vi "Util_CreateNIDrop.vi"(8 "error in (no error)":errorcluster) -> (0 "error out":errorcluster)   [LabVIEW 2011]
doc: "Runs the embedded application on a console located in the <B>Build Path</B> directory ."
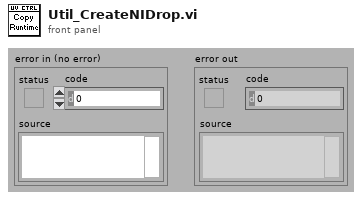
[diagram p1: front panel]
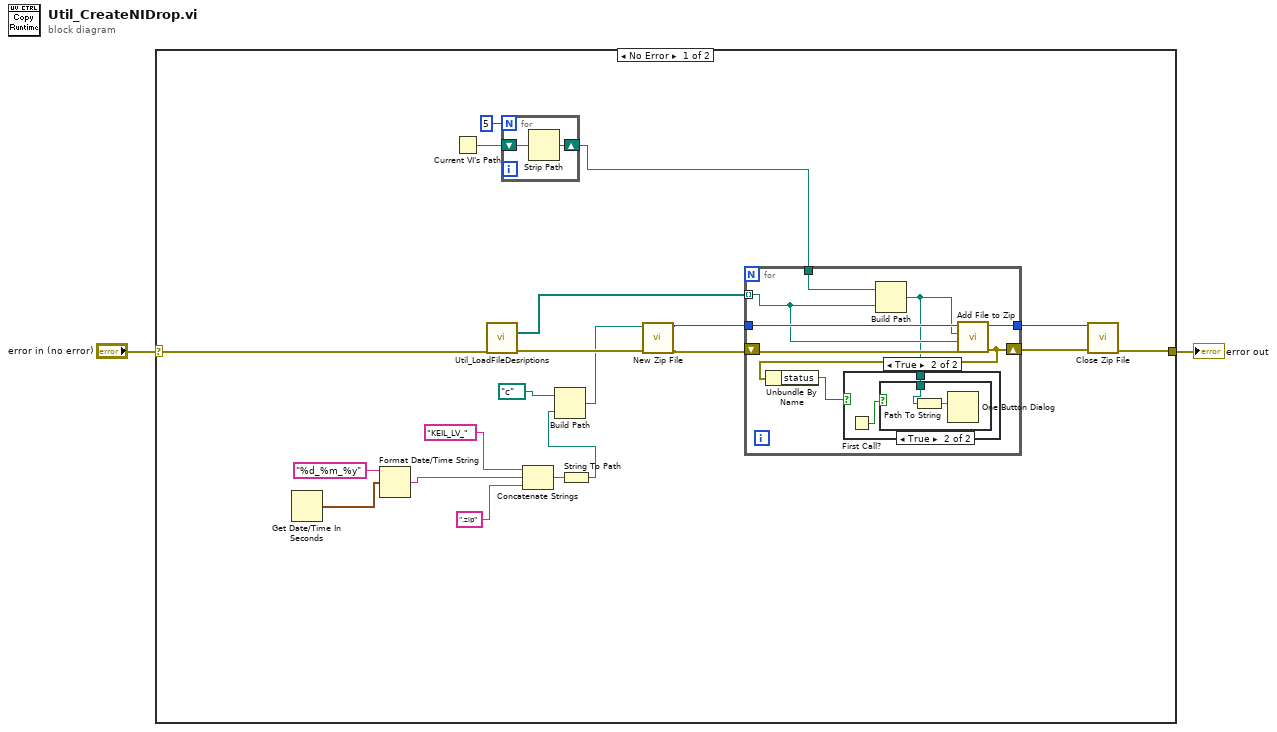
[diagram p0: block diagram]
diagram:
  n1 = case shown="No Error" "error in (no error)" {
    selector: "error in (no error)" -> [w16 w37]
    tunnel: [w10 w37] -> w1
    frame No Error {
      n2 = Get Date/Time In Seconds() -> (seconds since 1Jan1904=w22:timestamp)
      n3 = Format Date/Time String(time format string (%c)="%d_%m_%y", seconds (now)=w22) -> (date/time string=w8:string)  [unwired: 1 in]
      n4 = Current VI's Path() -> (path=w15:path)
      n5 = call "Util_LoadFileDesriptions.vi"("error in (no error)"=w16) -> ("Drop Files"=w17:path[], "error out"=w20:errorcluster)  [unwired: 9 in, 4 out]
      n6 = for {
        N: 5 -> [_]
        shift-right: [w23] -> w13
        shift-left: w15 -> [w24]
        n7 = Strip Path(path=w24) -> (stripped path=w23:path)  [unwired: 1 out]
      }
      n8 = Concatenate Strings("KEIL_LV_", w8, ".zip") -> (w6:string)
      n9 = String To Path(string=w6) -> (path=w3:path)
      n10 = Build Path(base path=path "c:/", name or relative path=w3) -> (appended path=w4:path)
      n11 = call <vilib>:"New Zip File.vi"("error in (no error)"=w20, "target"=w4) -> ("error out"=w19:errorcluster, "zip file out"=w18:i64)  [unwired: 3 in, 1 out]
      n12 = for {
        tunnel: w18 -> [w32]
        tunnel: w17 -> [w30] mode=indexing
        shift-right: [w27] -> w12
        shift-left: w19 -> [w31]
        tunnel: w13 -> [w29]
        tunnel: [w28] -> w11
        n13 = Build Path(base path=w29, name or relative path=w30) -> (appended path=w25:path)
        n14 = call <vilib>:"Add File to Zip.vi"("error in (no error)"=w31, "destination path in zip"=w30, "source file path"=w25, "zip file in"=w32) -> ("error out"=w27:errorcluster, "zip file out"=w28:i64)  [unwired: 6 in]
        n15 = Unbundle By Name(w27) -> ("status"=w26:bool)
        n16 = case shown="True" w26 {
          tunnel: w25 -> [_ w33]
          frame False {
          }
          frame True {
            n17 = First Call?() -> (First Call?: T/F=w34:bool)
            n18 = case shown="True" w34 {
              tunnel: w33 -> [_ w35]
              frame False {
              }
              frame True {
                n19 = Path To String(path=w35) -> (string=w36:string)
                n20 = One Button Dialog(message=w36) -> ()  [unwired: 1 in, 1 out]
              }
            }
          }
        }
      }
      n21 = call <vilib>:"Close Zip File.vi"("error in (no error)"=w12, "zip file in"=w11) -> ("error out"=w10:errorcluster)  [unwired: 5 in]
    }
    frame Error {
    }
  }
  "error out" <- w1
